vi "util-Analog-VoltageContinuousOutput-Change-For-Loop.vi"(0 "Channel(s)":tag="DAQ1/ao0", 1 "Output Array":T2(array[cluster])=[{"Waveform Type"=0, "Amplitude"=1.0, "Frequency"=10.0}] {"Frequency" format="%0.2p"; "Amplitude" format="%0.2p"; "Waveform Type" items=["Sine Wave", "Triangle Wave", "Square Wave", "Sawtooth Wave"]}, 2 "Duration(s)":dbl=5.0 caption="Delay Time (s)", 4 "Sample Rate":dbl=100000.0, 7 "error in":errorcluster) -> (20 "Waveform Graph":waveform(dbl)[](graph)=[{"t0"=timestamp(0 s since 1904-01-01), "dt"=0.001, "Y"=[]}], 27 "error out":errorcluster)   [LabVIEW 2020]
doc: "This example demonstrates how to continuously re-generate analog output data from a buffer in your computer's memory.\n\nRefer to your device documentation for pinouts and hardware capabilities."
uses:
  <vilib>/Utility/error.llb/DialogType.ctl
  <vilib>/DAQmx/write.llb/DAQmx Write (Analog Wfm 1Chan NSamp).vi
  <vilib>/Utility/file.llb/Read From Spreadsheet File (DBL).vi
  <vilib>/DAQmx/create/channels.llb/DAQmx Create Channel (AO-Voltage-Basic).vi
  <vilib>/DAQmx/configure/timing.llb/DAQmx Timing (Sample Clock).vi
  <vilib>/DAQmx/configure/trigger.llb/DAQmx Start Trigger (Digital Edge).vi
  <vilib>/DAQmx/configure/trigger.llb/DAQmx Start Trigger (Time).vi
  <vilib>/DAQmx/configure/trigger.llb/DAQmx Start Trigger (Analog Edge).vi
  <vilib>/DAQmx/miscellaneous.llb/DAQmx Fill In Error Info.vi
  <resource>/objmgr/daqmx.rc
  <vilib>/measure/NI_MABase.lvlib
panel:
  in  "Stop":bool
  out "all rows":dbl[](array[numeric])
  in  "Waveform File":path=path "D:/Generate analog waveform/Sine State 2.csv"
  in  "Trigger Type":T1(tab)
  in  "Digital Start Trigger Edge":i32(ring)=10280 caption="Edge" items=["Rising"=10280, "Falling"=10171]
  in  "Digital Start Trigger Source":tag="/Dev1/PFI0" caption="Source"
  in  "Digital Pause Trigger Pause When":i32(ring)=10192 caption="Pause When" items=["High"=10192, "Low"=10214]
  in  "Digital Pause Trigger Source":tag="/Dev1/PFI0" caption="Source"
  in  "Analog Start Trigger Level":dbl caption="Level" format="%0.2f"
  in  "Analog Start Trigger Hysteresis":dbl caption="Hysteresis" format="%.2f"
  in  "Analog Start Trigger Slope":i32(ring)=10280 caption="Slope" items=["Rising"=10280, "Falling"=10171]
  in  "Analog Start Trigger Source":string="APFI0" caption="Source"
  in  "Analog Pause Trigger Source":string="APFI0" caption="Source"
  in  "Analog Pause Trigger Pause When":i32(ring)=10093 caption="Pause When" items=["Above Level"=10093, "Below Level"=10107]
  in  "Analog Pause Trigger Level":dbl caption="Level" format="%.2f"
  in  "When":timestamp
  in  "Select Time\nManually":bool
  in  "Number of Samples":i32=10000
  in  "Sample Clock Source":tag="OnboardClock"
  in  "Max Voltage":dbl=5.0
  in  "Min Voltage":dbl=-5.0
  out "Actual Sample Rate":dbl=1000.0 format="%0.2f"
  # "Channel Settings"
  # "Output"
  # "Timing and\nBuffer Settings"
  # "Waveform Settings"
  # "Trigger Settings"
  # "The number of elements in the waveform array must equal the number of channels in the task."
  # "To enable triggers, select a tab above, and configure the settings.\n\nNot all hardware supports all trigger types. Refer to your device documentation for more information."
  # "This trigger type is not supported in output tasks. \n\nRefer to your device documentation for more information on which triggers are supported."
  # "This trigger type is not supported in output tasks. \n\nRefer to your device documentation for more information on which triggers are supported."
  # "If time is not manually set, task will begin after 10 seconds"
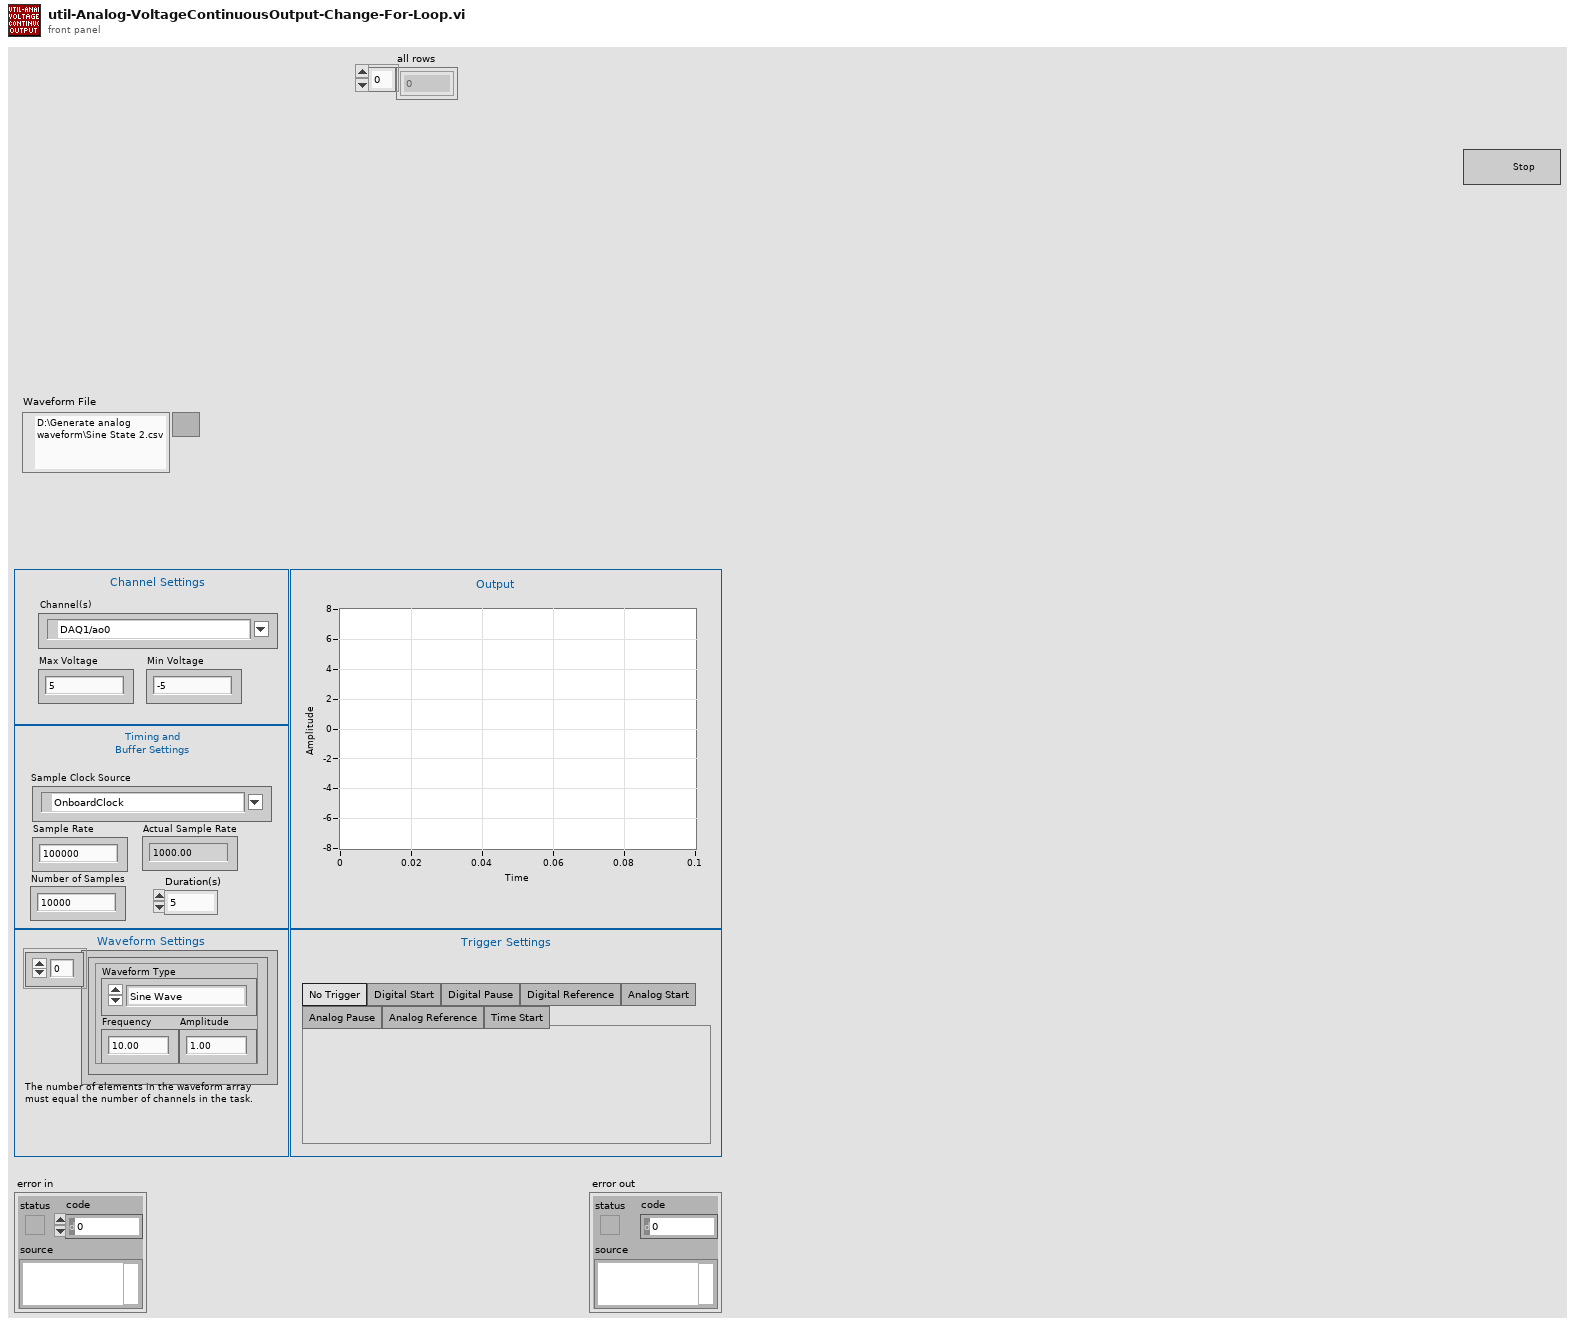
[diagram p1: front panel]
types:
  T1 = enum32{"No Trigger", "Digital Start", "Digital Pause", "Digital Reference", "Analog Start", "Analog Pause", "Analog Reference", "Time Start"}
  T2 = cluster{"Waveform Type":u16, "Amplitude":dbl, "Frequency":dbl}[]
  T3 = typedef "DialogType.ctl" = u16
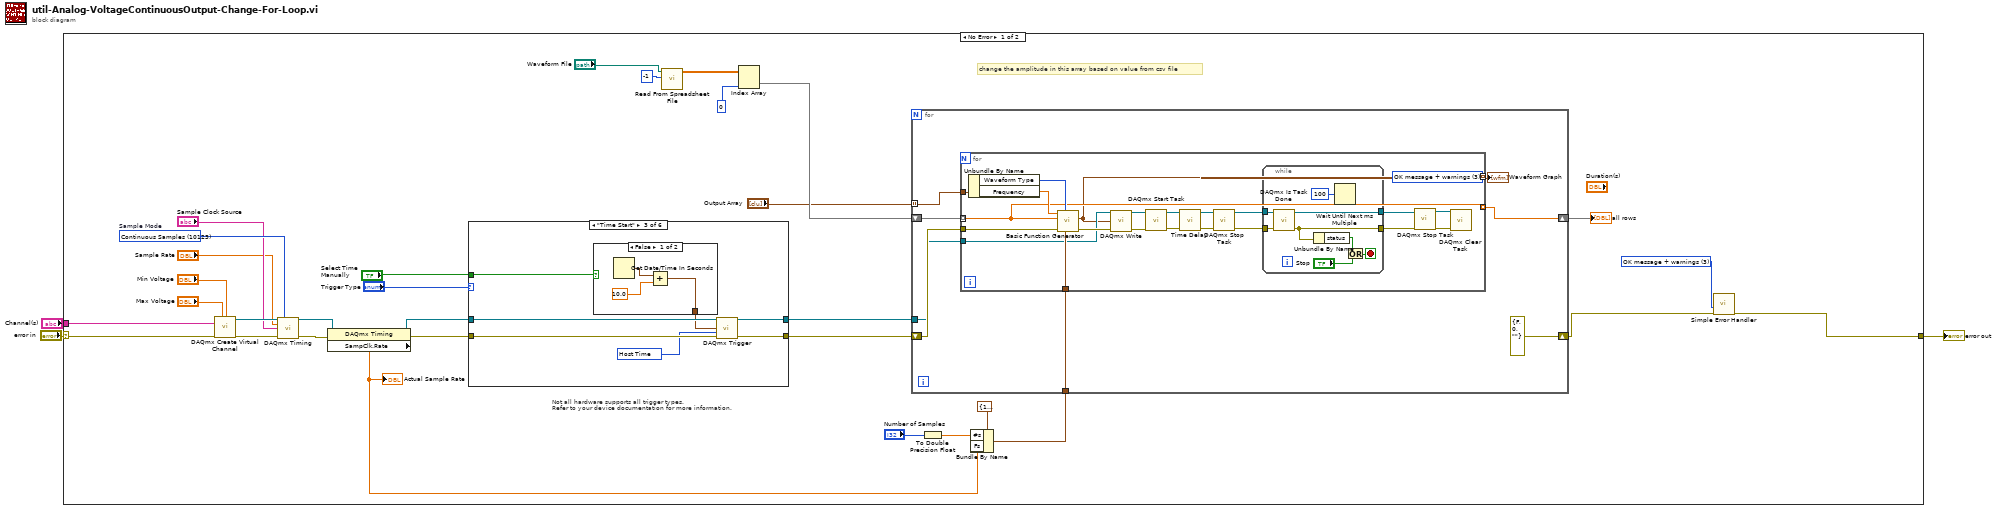
[diagram p0: block diagram]
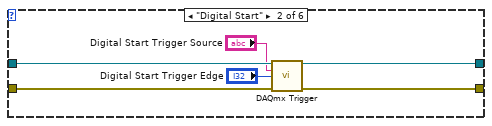
[diagram p3: hidden frame]
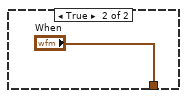
[diagram p4: hidden frame]
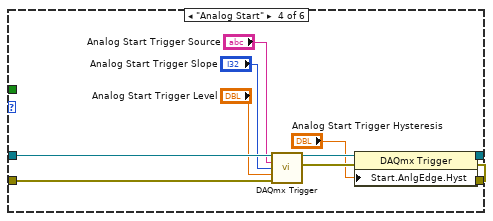
[diagram p5: hidden frame]
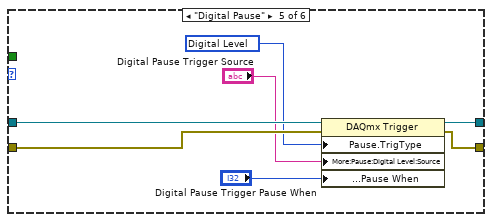
[diagram p6: hidden frame]
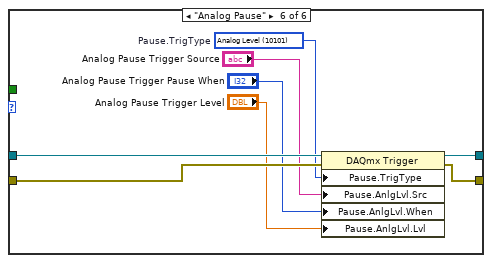
[diagram p7: hidden frame]
diagram:
  n1 = case shown="No Error" "error in" {
    selector: "error in" -> [w13 w116]
    tunnel: [w15 w116] -> w3
    tunnel: "Channel(s)" -> [w14 _]
    frame No Error {
      w21 = T3 3 items=["no dialog", "OK message", "continue or stop message", "OK message + warnings", "continue/stop + warnings"] ("type of dialog (OK msg:1)")
      w33 = 10123 items=["Finite Samples"=10178, "Continuous Samples"=10123, "Hardware Timed Single Point"=12522]  # Sample Mode
      # "change the amplitude in this array based on value from csv file"
      # "Not all hardware supports all trigger types.\nRefer to your device documentation for more information."
      n2 = call-poly <vilib>:"DAQmx Create Virtual Channel.vi"("maximum value"="Max Voltage", "minimum value"="Min Voltage", "physical channels"=w14, "error in"=w13) -> ("task out"=w31:refnum<k21>, "error out"=w32:errorcluster)  [unwired: 10 in]
      n3 = call-poly <vilib>:"DAQmx Timing.vi"("task/channels in"=w31, "sample mode"=w33, "rate"="Sample Rate", "source"="Sample Clock Source", "error in"=w32) -> ("task out"=w35:refnum<k21>, "error out"=w34:errorcluster)  [unwired: 9 in]
      n4 = property class="DAQmx Timing"(reference=w35, error in=w34) -> (reference out=w19:refnum<k21>, error out=w18:errorcluster, "SampClk.Rate"=w25:dbl)
      "Actual Sample Rate" <- w25
      n5 = case shown="\"Time Start\"" "Trigger Type" {
        tunnel: w19 -> [w73 w79 w86 w100 w107 w115]
        tunnel: w18 -> [w72 w78 w85 w99 w104 w112]
        tunnel: [w73 w77 w84 w97 w106 w114] -> w16
        tunnel: [w72 w76 w83 w96 w105 w113] -> w17
        tunnel: "Select Time\nManually" -> [_ _ w80 _ _ _]
        frame "No Trigger", Default {
        }
        frame "Digital Start" {
          n6 = call-poly <vilib>:"DAQmx Trigger.vi"("task/channels in"=w79, "source"="Digital Start Trigger Source", "edge"="Digital Start Trigger Edge", "error in"=w78) -> ("task out"=w77:refnum<k21>, "error out"=w76:errorcluster)  [unwired: 10 in]
        }
        frame "Time Start" {
          w82 = 16126 items=["Host Time"=16126, "I/O Device Time"=16127] ("timescale")
          n7 = case shown="False" w80 {
            tunnel: [w88 "When"] -> w81
            frame False {
              n8 = Get Date/Time In Seconds() -> (seconds since 1Jan1904=w89:timestamp)
              n9 = Add(x=w89, y=10.0) -> (x+y=w88:timestamp)
            }
            frame True {
            }
          }
          n10 = call-poly <vilib>:"DAQmx Trigger.vi"("task/channels in"=w86, "when"=w81, "timescale"=w82, "error in"=w85) -> ("task out"=w84:refnum<k21>, "error out"=w83:errorcluster)  [unwired: 10 in]
        }
        frame "Analog Start" {
          n11 = call-poly <vilib>:"DAQmx Trigger.vi"("task/channels in"=w100, "source"="Analog Start Trigger Source", "slope"="Analog Start Trigger Slope", "level"="Analog Start Trigger Level", "error in"=w99) -> ("task out"=w95:refnum<k21>, "error out"=w94:errorcluster)  [unwired: 9 in]
          n12 = property class="DAQmx Trigger"(reference=w95, error in=w94, "Start.AnlgEdge.Hyst"="Analog Start Trigger Hysteresis") -> (reference out=w97:refnum<k21>, error out=w96:errorcluster)
        }
        frame "Digital Pause" {
          w103 = 10152 items=["Analog Level"=10101, "Analog Window"=10103, "Digital Level"=10152, "Digital Pattern"=10398, "None"=10230] ("Pause.TrigType")
          n13 = property class="DAQmx Trigger"(reference=w107, error in=w104, "Pause.TrigType"=w103, "More:Pause:Digital Level:Source"="Digital Pause Trigger Source", "More:Pause:Digital Level:Pause When"="Digital Pause Trigger Pause When") -> (reference out=w106:refnum<k21>, error out=w105:errorcluster)
        }
        frame "Analog Pause" {
          w111 = 10101 items=["Analog Level"=10101, "Analog Window"=10103, "Digital Level"=10152, "Digital Pattern"=10398, "None"=10230]  # Pause.TrigType
          n14 = property class="DAQmx Trigger"(reference=w115, error in=w112, "Pause.TrigType"=w111, "Pause.AnlgLvl.Src"="Analog Pause Trigger Source", "Pause.AnlgLvl.When"="Analog Pause Trigger Pause When", "Pause.AnlgLvl.Lvl"="Analog Pause Trigger Level") -> (reference out=w114:refnum<k21>, error out=w113:errorcluster)
        }
      }
      n15 = call-poly <vilib>:"Read From Spreadsheet File.vi"("number of rows (all:-1)"=-1, "file path (dialog if empty)"="Waveform File") -> ("all rows"=w10:dbl[][])  [unwired: 5 in, 4 out]
      n16 = Index Array(array=w10, index (col)=0 ("disabled index (col)")) -> (element=w7:dbl[])  [unwired: 1 in]
      n17 = To Double Precision Float(number="Number of Samples") -> (double precision float=w23:dbl)
      n18 = Bundle By Name(cluster=cluster{"Fs":dbl, "#s":dbl} {"Fs"=1000.0, "#s"=1000.0} ("sampling info"), "#s"=w23, "Fs"=w25) -> (w24:cluster{"Fs":dbl, "#s":dbl})
      n19 = for {
        tunnel: w24 -> [w43]
        tunnel: "Output Array" -> [w39] mode=indexing
        shift-right: [w38] -> w5
        shift-left: w7 -> [w40]
        tunnel: w16 -> [w37]
        shift-right: [errorcluster {"status"=FALSE, "code"=0, "source"=""} ("error out")] -> w4
        shift-left: w17 -> [w41]
        n20 = for {
          tunnel: w41 -> [w63]
          tunnel: w43 -> [w62]
          tunnel: [w44] -> w42 mode=indexing
          tunnel: w39 -> [w59]
          tunnel: w40 -> [w55] mode=indexing
          tunnel: [w55] -> w38 mode=indexing
          tunnel: w37 -> [w56]
          (unwired) T3 3 items=["no dialog", "OK message", "continue or stop message", "OK message + warnings", "continue/stop + warnings"] ("type of dialog (OK msg:1)")
          n21 = Unbundle By Name(w59) -> ("Waveform Type"=w61:u16, "Frequency"=w60:dbl)
          n22 = call <vilib>:"Basic Function Generator.vi"("sampling info"=w62, "signal type"=w61, "error in (no error)"=w63, "amplitude"=w55, "frequency"=w60) -> ("error out"=w57:errorcluster, "signal out"=w44:waveform(dbl))  [unwired: 4 in, 1 out]
          n23 = call-poly <vilib>:"DAQmx Write.vi"("task/channels in"=w56, "data"=w44, "error in"=w57) -> ("task out"=w54:refnum<k21>, "error out"=w58:errorcluster)  [unwired: 10 in, 1 out]
          n24 = call <vilib>:"DAQmx Start Task.vi"("task/channels in"=w54, "error in"=w58) -> ("task out"=w53:refnum<k21>, "error out"=w52:errorcluster)  [unwired: 12 in]
          n25 = call "Time Delay"("error in (no error)"=w52) -> ("error out"=w51:errorcluster)  [unwired: 10 in]
          n26 = call <vilib>:"DAQmx Stop Task.vi"("task/channels in"=w53, "error in"=w51) -> ("task out"=w46:refnum<k21>, "error out"=w45:errorcluster)  [unwired: 12 in]
          n27 = while {
            tunnel: w46 -> [w71]
            tunnel: w45 -> [w70]
            tunnel: [w67] -> w47
            tunnel: [w68] -> w48
            stop <- w69 stop-if-true
            n28 = call <vilib>:"DAQmx Is Task Done.vi"("task/channels in"=w71, "error in"=w70) -> ("task out"=w68:refnum<k21>, "error out"=w67:errorcluster)  [unwired: 11 in, 1 out]
            n29 = Unbundle By Name(w67) -> ("status"=w66:bool)
            n30 = Wait Until Next ms Multiple(millisecond multiple=u32 100) -> ()  [unwired: 1 out]
            n31 = Or(x=w66, y="Stop") -> (x .or. y?=w69:bool)
          }
          n32 = call <vilib>:"DAQmx Stop Task.vi"("task/channels in"=w48, "error in"=w47) -> ("task out"=w50:refnum<k21>, "error out"=w49:errorcluster)  [unwired: 12 in]
          n33 = call <vilib>:"DAQmx Clear Task.vi"("task in"=w50, "error in"=w49) -> ()  [unwired: 13 in, 1 out]
        }
        "Waveform Graph" <- w42
      }
      "all rows" <- w5
      n34 = call <vilib>:"Simple Error Handler.vi"("type of dialog (OK msg:1)"=w21, "error in (no error)"=w4) -> ("error out"=w15:errorcluster)  [unwired: 3 in, 4 out]
    }
    frame Error {
    }
  }
  "error out" <- w3
